vi "LWXPS_GroupSpinParametersGet.vi"(8 "LabVIEW error IN":errorcluster, 10 "Group Name":string, 11 "XPS Reference IN":refnum<k24>) -> (0 "XPS Error String":string, 1 "Acceleration":dbl, 2 "Velocity":dbl, 3 "Returned error code":i32, 4 "LabVIEW error OUT":errorcluster, 5 "XPS Reference OUT":refnum<k24>)   [LabVIEW 2014]
uses:
  D:/XPSQ8_LabView_Library/Development/Source/Dll/Newport.XPS.CommandInterface.dll
  Dll/Newport.XPS.CommandInterface.dll
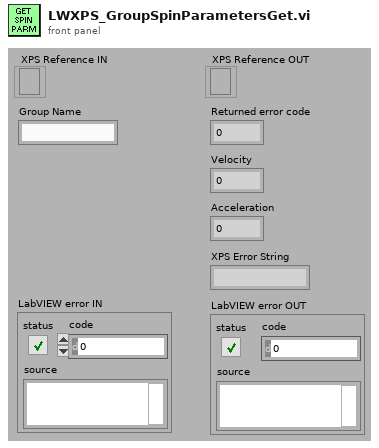
[diagram p1: front panel]
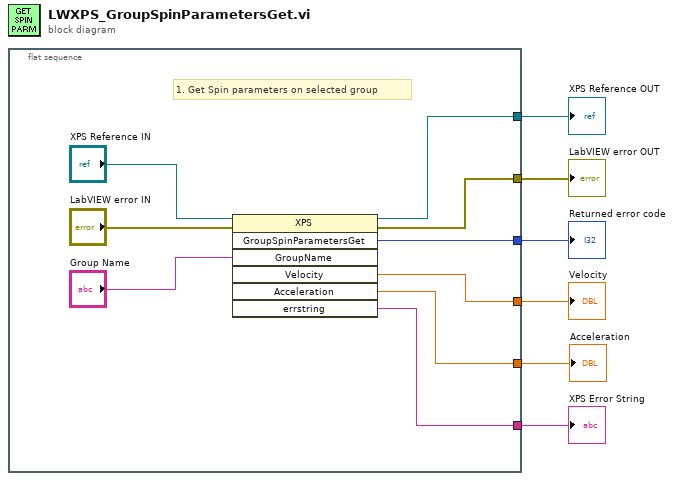
[diagram p0: block diagram]
diagram:
  n1 = flat-sequence {
    tunnel: [w11] -> w6
    tunnel: [w13] -> w5
    tunnel: [w14] -> w4
    tunnel: [w7] -> w1
    tunnel: [w9] -> w2
    tunnel: [w8] -> w3
    frame #0 {
      # "1. Get Spin parameters on selected group"
      n2 = invoke class="XPS" method="GroupSpinParametersGet"(reference="XPS Reference IN", error in="LabVIEW error IN", "GroupName"="Group Name") -> (reference out=w11:refnum<k24>, error out=w13:errorcluster, "GroupSpinParametersGet"=w14:i32, "Velocity"=w9:dbl, "Acceleration"=w7:dbl, "errstring"=w8:string)  [unwired: 4 in, 1 out]
    }
  }
  "XPS Reference OUT" <- w6
  "LabVIEW error OUT" <- w5
  "Returned error code" <- w4
  "XPS Error String" <- w3
  "Velocity" <- w2
  "Acceleration" <- w1
